vi "Calculate A F Q.vi"(10 "Camera":T2, 11 "Screen Dimensions":T1) -> (1 "q":sgl, 2 "f":sgl, 3 "Aspect Ratio":sgl)   [LabVIEW 2020, in "3D (FPGA).lvlib"]
uses:
  3D (FPGA).lvlib
  Camera.ctl
  Raster/Rectangle Dimensions.ctl
  Raster/Raster (FPGA).lvlib
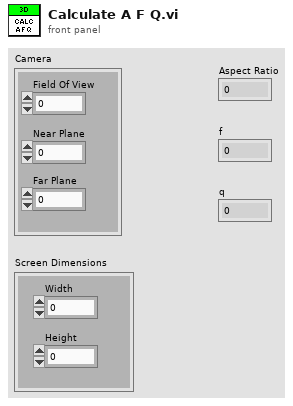
[diagram p1: front panel]
types:
  T1 = typedef "Raster (FPGA).lvlib/Rectangle Dimensions.ctl" = cluster{"Width":u32, "Height":u32}
  T2 = typedef "3D (FPGA).lvlib/Camera.ctl" = cluster{"Field Of View":sgl, "Near Plane":sgl, "Far Plane":sgl}
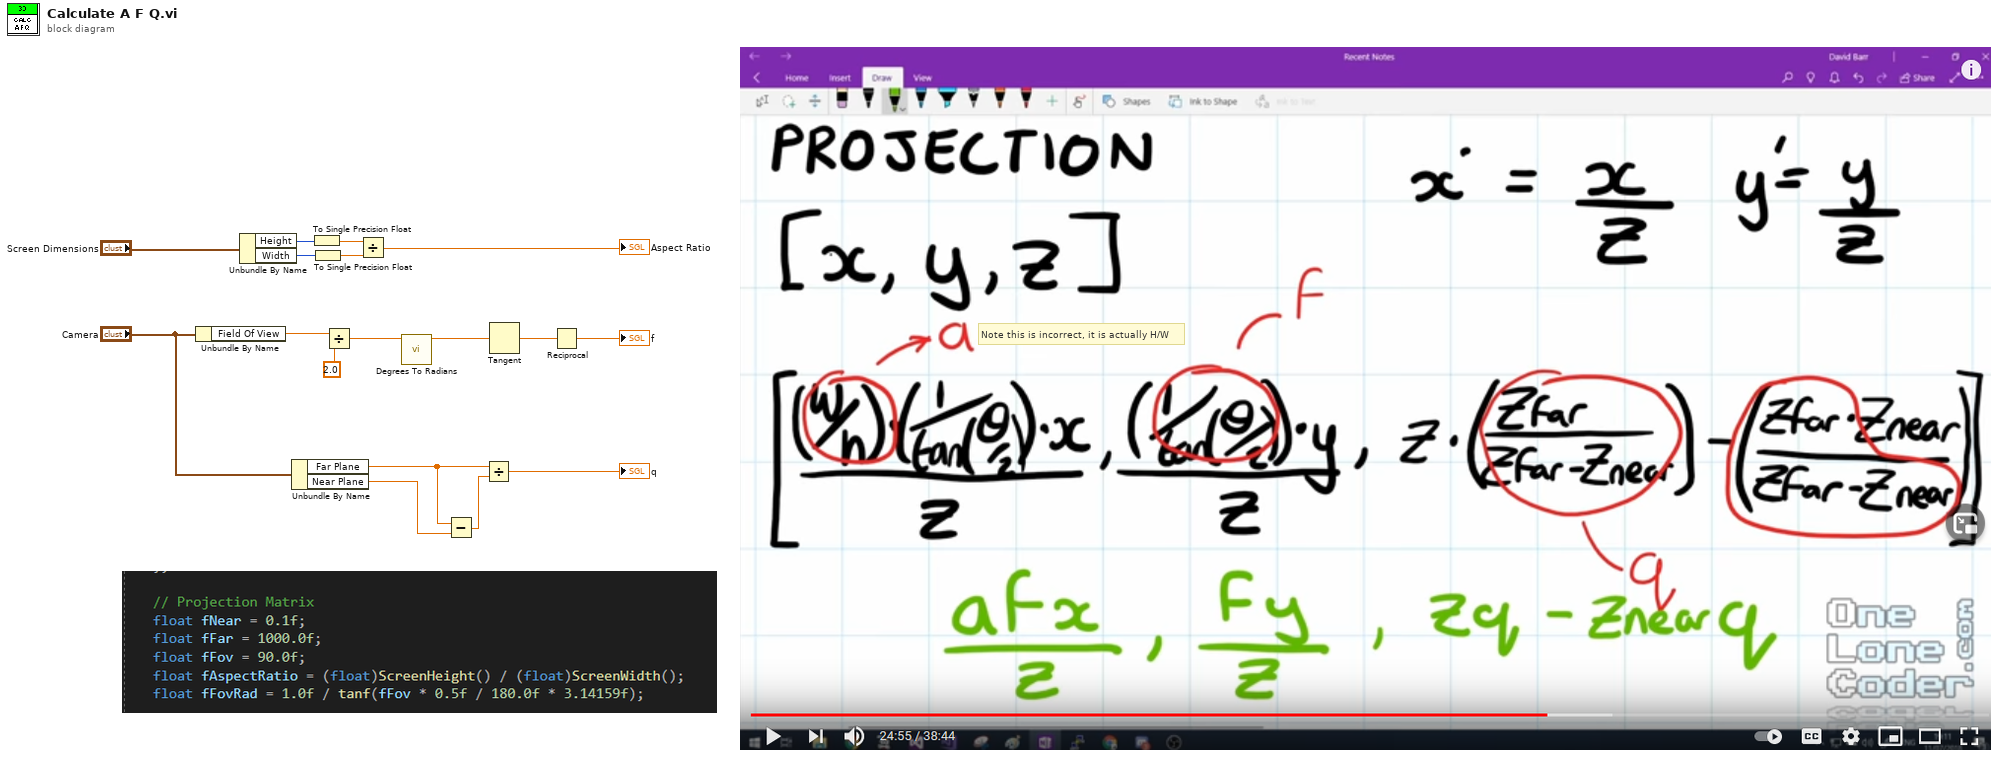
[diagram p0: block diagram]
diagram:
  # "Note this is incorrect, it is actually H/W"
  n1 = Unbundle By Name("Camera") -> ("Field Of View"=w10:sgl)
  n2 = Unbundle By Name("Screen Dimensions") -> ("Height"=w16:u32, "Width"=w15:u32)
  n3 = Unbundle By Name("Camera") -> ("Far Plane"=w7:sgl, "Near Plane"=w6:sgl)
  n4 = To Single Precision Float(number=w16) -> (single precision float=w14:sgl)
  n5 = To Single Precision Float(number=w15) -> (single precision float=w13:sgl)
  n6 = Divide(x=w10, y=sgl 2.0) -> (x/y=w2:sgl)
  n7 = Divide(x=w14, y=w13) -> (x/y=→"Aspect Ratio":sgl)
  n8 = call "Degrees To Radians.vi"("Angle (°)"=w2) -> ("Angle (rad)"=w1:sgl)  [unwired: 10 in]
  n9 = Subtract(x=w7, y=w6) -> (x-y=w5:sgl)
  n10 = Divide(x=w7, y=w5) -> (x/y=→"q":sgl)
  n11 = Tangent(1:w1) -> (0:w9:sgl)
  n12 = Reciprocal(x=w9) -> (1/x=→"f":sgl)
